vi "SLSC Enable Buttons.vi"(8 "error in (no error)":errorcluster, 11 "data":T1) -> ()   [LabVIEW 2015, in "SLSC EDS System Explorer.lvlib"]
uses:
  System Explorer/SLSC EDS System Explorer.lvlib
  SLSC EDS API/JSON parsing/EDSjsonStructure.ctl
  SLSC EDS API/JSON parsing/enum.ctl
  SLSC EDS API/JSON parsing/property.ctl
  SLSC EDS API/JSON parsing/command.ctl
  SLSC EDS API/JSON parsing/scale.ctl
  SLSC EDS API/JSON parsing/physicalChannel.ctl
  SLSC EDS API/JSON parsing/register.ctl
  <vilib>/NI VeriStand/Custom Device API/Custom Device API.lvlib
panel:
  # "not working\nregisterMap->registers->initialValue"
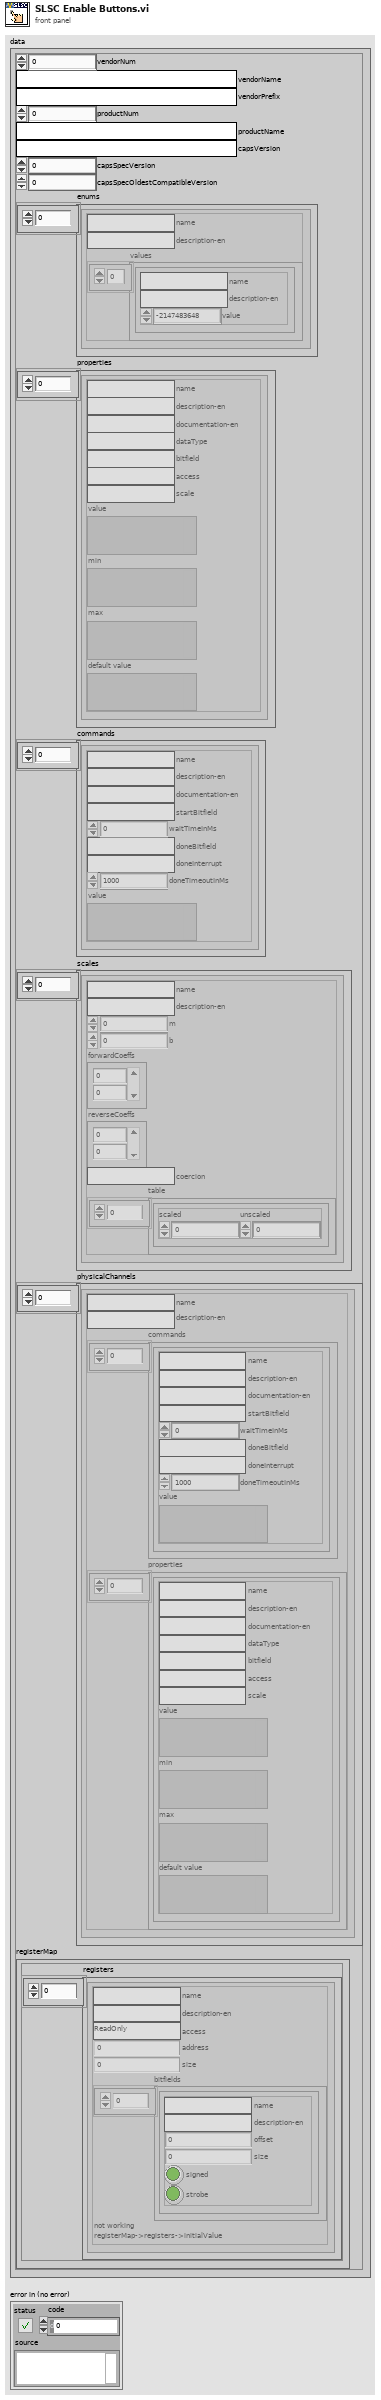
[diagram p1: front panel]
types:
  T1 = typedef "EDSjsonStructure.ctl" = cluster{"vendorNum":u32, "vendorName":string, "vendorPrefix":string, "productNum":u32, "productName":string, "capsVersion":string, "capsSpecVersion":u32, "capsSpecOldestCompatibleVersion":u32, "enums":T2[], "properties":T3[], "commands":T4[], "scales":T5[], "physicalChannels":T6[], "registerMap":cluster{"registers":T7[]}}
  T2 = typedef "enum.ctl" = cluster{"name":string, "description-en":string, "values":cluster{"name":string, "description-en":string, "value":i32}[]}
  T3 = typedef "property.ctl" = cluster{"name":string, "description-en":string, "documentation-en":string, "dataType":string, "bitfield":string, "access":string, "scale":string, "value":variant, "min":variant, "max":variant, "default value":variant}
  T4 = typedef "command.ctl" = cluster{"name":string, "description-en":string, "documentation-en":string, "startBitfield":string, "waitTimeInMs":i32, "doneBitfield":string, "doneInterrupt":string, "doneTimeoutInMs":i32, "value":variant}
  T5 = typedef "scale.ctl" = cluster{"name":string, "description-en":string, "m":dbl, "b":dbl, "forwardCoeffs":dbl[], "reverseCoeffs":dbl[], "coercion":string, "table":cluster{"scaled":dbl, "unscaled":dbl}[]}
  T6 = typedef "physicalChannel.ctl" = cluster{"name":string, "description-en":string, "commands":T4[], "properties":T3[]}
  T7 = typedef "register.ctl" = cluster{"name":string, "description-en":string, "access":string, "address":u32, "size":u32, "bitfields":cluster{"name":string, "description-en":string, "offset":u32, "size":u32, "signed":bool, "strobe":bool}[]}
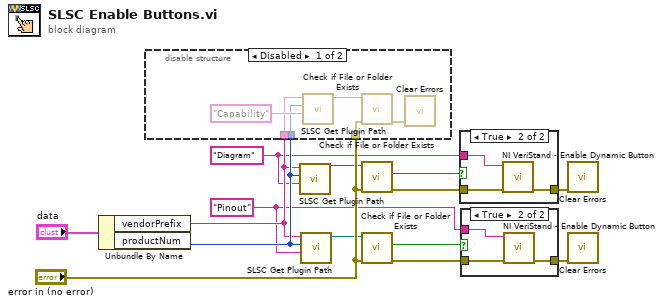
[diagram p0: block diagram]
diagram:
  w4 = "Diagram" ("Type")
  w6 = "Pinout" ("Type")
  n1 = Unbundle By Name("data") -> ("vendorPrefix"=w12:string, "productNum"=w13:u32)
  n2 = disable-structure shown="Disabled" {
    disable-tunnel: "error in (no error)" -> [w19 _]
    disable-tunnel: w13 -> [w16 _]
    disable-tunnel: w12 -> [w15 _]
    frame Disabled {
      n3 = call "SLSC Get Plugin Path.vi"("Type"="Capability", "number"=w16, "Vendor Prefix"=w15) -> ("appended path"=w18:path)  [unwired: 8 in]
      n4 = call <vilib>:"Check if File or Folder Exists.vi"("error in (no error)"=w19, "path"=w18) -> ("error out"=w20:errorcluster)  [unwired: 7 in, 2 out]
      n5 = call <vilib>:"Clear Errors.vi"("error in (no error)"=w20) -> ()  [unwired: 1 in, 6 out]
    }
    frame Enabled {
    }
  }
  n6 = call "SLSC Get Plugin Path.vi"("Type"=w4, "number"=w13, "Vendor Prefix"=w12) -> ("appended path"=w2:path)  [unwired: 8 in]
  n7 = call "SLSC Get Plugin Path.vi"("Type"=w6, "number"=w13, "Vendor Prefix"=w12) -> ("appended path"=w3:path)  [unwired: 8 in]
  n8 = call <vilib>:"Check if File or Folder Exists.vi"("error in (no error)"="error in (no error)", "path"=w2) -> ("error out"=w8:errorcluster, "file or folder exists?"=w5:bool)  [unwired: 7 in, 1 out]
  n9 = call <vilib>:"Check if File or Folder Exists.vi"("error in (no error)"="error in (no error)", "path"=w3) -> ("error out"=w9:errorcluster, "file or folder exists?"=w7:bool)  [unwired: 7 in, 1 out]
  n10 = case shown="True" w5 {
    tunnel: w4 -> [_ w24]
    tunnel: w8 -> [w21 w23]
    tunnel: [w21 w22] -> w10
    frame False {
    }
    frame True {
      n11 = call <vilib>:"NI VeriStand - Enable Dynamic Button.vi"("error in (no error)"=w23, "Button ID"=w24) -> ("error out"=w22:errorcluster)  [unwired: 9 in]
    }
  }
  n12 = case shown="True" w7 {
    tunnel: w6 -> [_ w28]
    tunnel: w9 -> [w25 w27]
    tunnel: [w25 w26] -> w11
    frame False {
    }
    frame True {
      n13 = call <vilib>:"NI VeriStand - Enable Dynamic Button.vi"("error in (no error)"=w27, "Button ID"=w28) -> ("error out"=w26:errorcluster)  [unwired: 9 in]
    }
  }
  n14 = call <vilib>:"Clear Errors.vi"("error in (no error)"=w10) -> ()  [unwired: 1 in, 6 out]
  n15 = call <vilib>:"Clear Errors.vi"("error in (no error)"=w11) -> ()  [unwired: 1 in, 6 out]
